vi "False.vi"() -> (0 "error out":errorcluster)   [LabVIEW 2017, in "Transparent Assertions.Tests.lvlib" / "Assert True.lvlib"]
uses:
  Assert True.lvlib
  src/Transparent Assertions/Transparent Assertions.lvlib
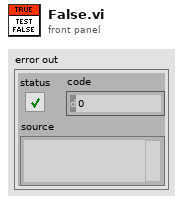
[diagram p1: front panel]
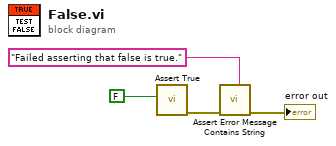
[diagram p0: block diagram]
diagram:
  n1 = call "Assert True.vi"("Condition"=FALSE) -> ("error out"=w3:errorcluster)  [unwired: 10 in]
  n2 = call "Assert Error Message Contains String.vi"("Expected"="Failed asserting that false is true." ("y"), "error in (no error)"=w3) -> ("error out"=→"error out":errorcluster)  [unwired: 9 in]
